vi "tsapp_log_win32.vi"(8 "错误输入（无错误）":errorcluster, 10 "ALevel":i32, 11 "AStr":string) -> (0 "错误输出":errorcluster, 3 "tsapp_log":i32)   [LabVIEW 2010]
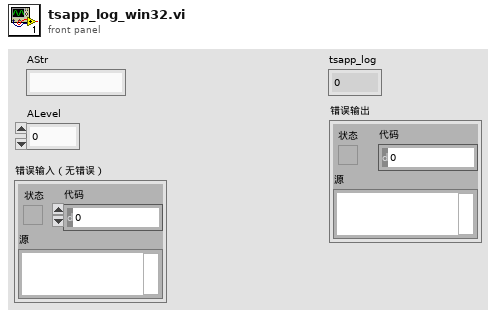
[diagram p1: front panel]
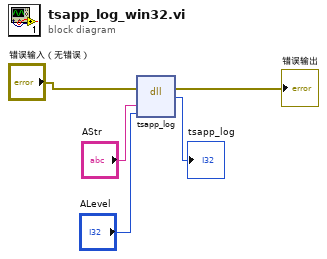
[diagram p0: block diagram]
diagram:
  n1 = dll-call lib="PTH1`abs DLabviewWorkSpace海卓项目资料\tHaiDriverBottomLevelTS_CANDriveTSMaster.dll" fn="tsapp_log"(error in="错误输入（无错误）", "AStr"="AStr", "ALevel"="ALevel") -> (error out=→"错误输出":errorcluster, "tsapp_log"=→"tsapp_log":i32)  [unwired: 4 in, 1 out]
